vi "Begin.vi"(8 "error in":errorcluster) -> (0 "error out":errorcluster)   [LabVIEW 2015]
doc: "Called before other user functions, this VI is expected to open initial I/O refnums, load in file data, and do all program initialization. Notice that the <B>error out</B> terminal is simply used for data flow. Wiring it to other structures or subVIs ensures that this VI runs first."
uses:
  <vilib>/Rock Robotics/WPI/DriverStation/WPI_DriverStationRobotMode2.ctl
  <vilib>/Rock Robotics/WPI/Joystick/WPI_JoystickDeviceEnum.ctl
  <vilib>/Rock Robotics/SystemInterfaces/DIO/FPGA_DIOPWMChannel.ctl
  <vilib>/Rock Robotics/WPI/SafetyOutput/WPI_SafetyOutputConfigMenu.ctl
  <vilib>/Rock Robotics/WPI/Solenoid/WPI_SolenoidChannel.ctl
  <vilib>/Rock Robotics/SystemInterfaces/DIO/FPGA_DIOChannel.ctl
  <vilib>/Rock Robotics/WPI/Encoder/WPI_EncoderType.ctl
  <vilib>/Rock Robotics/SystemInterfaces/AI/FPGA_AIChannel.ctl
  <vilib>/Rock Robotics/SystemInterfaces/spilib/spi_bus.ctl
  Robot Global Data.vi
  <vilib>/Rock Robotics/WPI/Counter/WPI_CounterDigitalInputToDigitalSource.vi
  <vilib>/Rock Robotics/WPI/Solenoid/WPI_SolenoidOpenSingle.vi
  <vilib>/Rock Robotics/WPI/MotorControl/WPI_MotorControlOpen VictorSP.vi
  <vilib>/Rock Robotics/WPI/Utilities/WPI_GetSetVariantRefNum.vi
  navX Library v2/IO/Open/Z900_navX_Open_SPI.vi
  <vilib>/Rock Robotics/WPI/RobotDrive/WPI_RobotDriveOpen2MotorWithVictorSP.vi
  navX Library v2/navX Library v2.lvlib
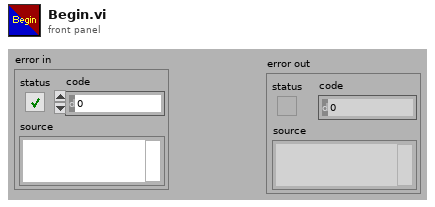
[diagram p1: front panel]
types:
  T1 = typedef "WPI_SolenoidChannel.ctl" = enum8{"Solenoid 0", "Solenoid 1", "Solenoid 2", "Solenoid 3", "Solenoid 4", "Solenoid 5", "Solenoid 6", "Solenoid 7", "Invalid"}
  T2 = typedef "FPGA_DIOPWMChannel.ctl" = enum8{"PWM 0", "PWM 1", "PWM 2", "PWM 3", "PWM 4", "PWM 5", "PWM 6", "PWM 7", "PWM 8", "PWM 9", "PWM MXP 0", "PWM MXP 1", "PWM MXP 2", "PWM MXP 3", "PWM MXP 4", "PWM MXP 5", "PWM MXP 6", "PWM MXP 7", "PWM MXP 8", "PWM MXP 9", "Invalid"}
  T3 = typedef "FPGA_DIOChannel.ctl" = enum8{"DIO 0", "DIO 1", "DIO 2", "DIO 3", "DIO 4", "DIO 5", "DIO 6", "DIO 7", "DIO 8", "DIO 9", "DIO MXP 0", "DIO MXP 1", "DIO MXP 2", "DIO MXP 3", "DIO MXP 4", "DIO MXP 5", "DIO MXP 6", "DIO MXP 7", "DIO MXP 8", "DIO MXP 9", "DIO MXP 10", "DIO MXP 11", "DIO MXP 12", "DIO MXP 13", "DIO MXP 14", "DIO MXP 15", "Invalid"}
  T4 = typedef "spi_bus.ctl" = enum16{"SPI On-Board, CS0", "SPI On-Board, CS1", "SPI On-Board, CS2", "SPI On-Board, CS3", "SPI MXP", "Invalid"}
  T5 = typedef "FPGA_AIChannel.ctl" = enum8{"AI 0", "AI 1", "AI 2", "AI 3", "AI MXP 0", "AI MXP 1", "AI MXP 2", "AI MXP 3", "Invalid"}
  T6 = typedef "WPI_JoystickDeviceEnum.ctl" = enum16{"USB 0", "USB 1", "USB 2", "USB 3", "USB 4", "USB 5"}
  T7 = typedef "WPI_EncoderType.ctl" = enum16{"1x", "2x", "4x"}
  T8 = typedef "WPI_SafetyOutputConfigMenu.ctl" = enum16{"Enable", "Disable"}
  T9 = typedef "WPI_DriverStationRobotMode2.ctl" = enum16{"Autonomous Disabled", "Autonomous Enabled", "Teleop Disabled", "Teleop Enabled", "Disconnected", "Finish", "Test Disabled", "Test Enabled", "Emergency Stopped"}
  T10 = typedef "WPI_MotorControlDeviceRef.ctl" = cluster{"DeviceStatus":errorcluster, "Type":T11, "PWM":cluster{"PWM Channel":T2, "DeadBand":T12}, "CAN":cluster{"Device Number":u8, "Control Mode":T13, "Semaphore":T14, "Max Vout":dbl, "TalonSRX Control Mode":T15}, "Invert":bool}
  T11 = typedef "WPI_MotorControlType.ctl" = enum16{"PWM", "CAN", "CANTalonSRX"}
  T12 = typedef "WPI_PWMDeadband.ctl" = cluster{"Name":string, "maxPositivePwm":i32, "minPositivePwm":i32, "centerPwm":i32, "maxNegativePwm":i32, "minNegativePwm":i32, "angularRange":u16}
  T13 = typedef "WPI_CANJaguar_ControlMode.ctl" = enum8{"Percent VBus", "Current", "Speed", "Position", "Voltage"}
  T14 = typedef "Semaphore RefNum" = refnum<k1>
  T15 = typedef "WPI_CANTalonSRX_APIControlMode.ctl" = enum8{"Percent VBus", "Speed", "Position", "Slave", "Unchanged / Invalid", "Voltage Compensation", "Current", "Motion Profile"}
  T16 = typedef "WPI_CompressorDevRef.ctl" = cluster{"DevStatus":errorcluster, "Pneumatics Control Module":u8}
  T17 = typedef "WPI_DigitalInputDevRef.ctl" = cluster{"DevStatus":errorcluster, "DIO Channel":T3}
  T18 = typedef "WPI_RobotDriveDevRef.ctl" = cluster{"DevStatus":errorcluster, "Motors[]":T10[], "Square Inputs":bool, "Max Output":dbl}
  T19 = typedef "WPI_JoystickDevRef.ctl" = cluster{"Device":T6}
  T20 = typedef "FPGA_CounterEncoderSourceConvertionLVSourceType.ctl" = cluster{"DevStatus":errorcluster, "AnalogTriggerMode?":bool, "DigitalMode":cluster{"DIO Channel":T21}, "AnalogTriggerMode":cluster{"AnalogTriggerIndex":T22, "OutputType":T23}}
  T21 = typedef "FPGA_DIODigitalSourceChannel.ctl" = enum8{"DIO 0", "DIO 1", "DIO 2", "DIO 3", "DIO 4", "DIO 5", "DIO 6", "DIO 7", "DIO 8", "DIO 9", "DIO MXP 0", "DIO MXP 1", "DIO MXP 2", "DIO MXP 3", "DIO MXP 4", "DIO MXP 5", "DIO MXP 6", "DIO MXP 7", "DIO MXP 8", "DIO MXP 9", "DIO MXP 10", "DIO MXP 11", "DIO MXP 12", "DIO MXP 13", "DIO MXP 14", "DIO MXP 15", "Disabled"}
  T22 = typedef "FPGA_AnalogTriggerIndex.ctl" = enum8{"Trig 0", "Trig 1", "Trig 2", "Trig 3", "Trig 4", "Trig 5", "Trig 6", "Trig 7", "Invalid"}
  T23 = typedef "FPGA_AnalogTriggerOutType.ctl" = enum16{"InWindow", "TriggerState", "Rising", "Falling"}
  T24 = typedef "navX Library v2.lvlib/Z900_navX_DeviceTypeDef.ctl" = cluster{"Interface":cluster{"Protocol":T25, "Update Rate (4Hz-60Hz)":u8, "navX Open TypeDef":variant}, "Notify Packet":refnum<notifier>, "Loop VI Refnum":refnum<vi>, "Ready to Close Occurrence Refnum":refnum<k4>}
  T25 = typedef "navX Library v2.lvlib/Z900_navX_ProtocolTypeDef.ctl" = enum16{"SERIAL", "I2C", "SPI"}
  T26 = typedef "WPI_AnalogChannelDevRef.ctl" = cluster{"DevStatus":errorcluster, "Analog Channel":T5}
  T27 = typedef "WPI_PotentiometerDevRef.ctl" = cluster{"DevStatus":errorcluster, "Analog Channel":T5, "Invert Output":bool}
  T28 = typedef "WPI_EncoderDevRef.ctl" = cluster{"DevStatus":errorcluster, "EncoderIndex":T29, "CounterIndex":T30, "DistancePerCount":dbl, "Decoding Type":T7}
  T29 = typedef "FPGA_EncoderIdx.ctl" = enum8{"Enc 0", "Enc 1", "Enc 2", "Enc 3", "Enc 4", "Enc 5", "Enc 6", "Enc 7", "Invalid"}
  T30 = typedef "FPGA_CounterCtrSystemIndex.ctl" = enum8{"Ctr 0", "Ctr 1", "Ctr 2", "Ctr 3", "Ctr 4", "Ctr 5", "Ctr 6", "Ctr 7", "Invalid"}
  T31 = typedef "WPI_SolenoidDevRef.ctl" = cluster{"DevStatus":errorcluster, "Pneumatics Control Module":u8, "Forward Solenoid Channel":T1, "Reverse Solenoid Channel":T1}
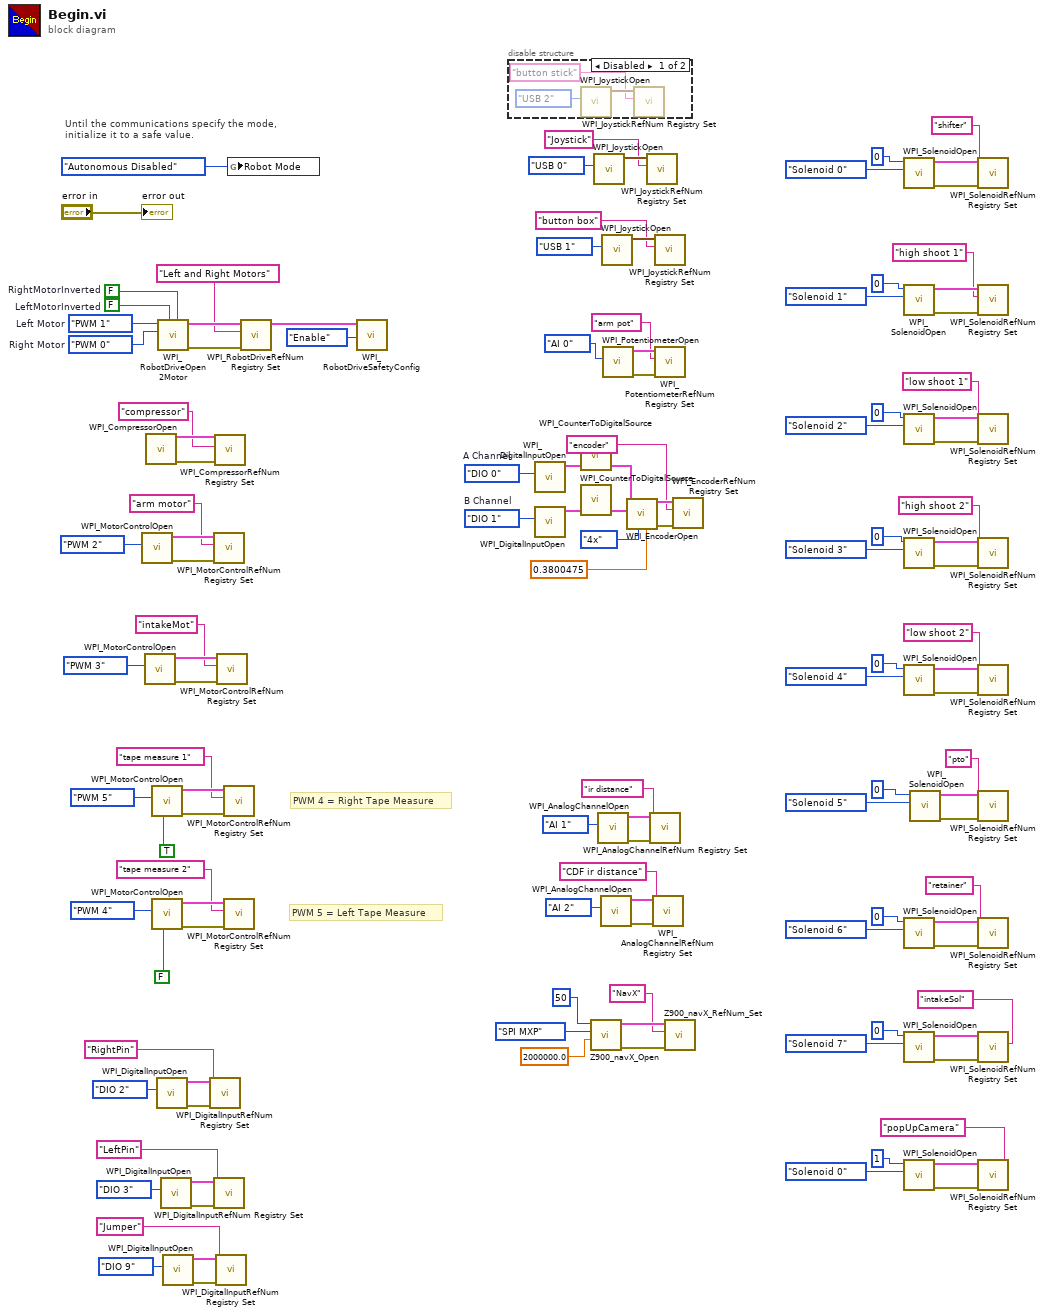
[diagram p0: block diagram]
diagram:
  w103 = FPGA_DIOChannel."DIO 1"  # B Channel
  w102 = FPGA_DIOChannel."DIO 0"  # A Channel
  w113 = FPGA_DIOPWMChannel."PWM 0"  # Right Motor
  w114 = FPGA_DIOPWMChannel."PWM 1"  # Left Motor
  w118 = FALSE  # LeftMotorInverted
  w119 = FALSE  # RightMotorInverted
  # "PWM 5 = Left Tape Measure"
  # "PWM 4 = Right Tape Measure"
  # "Until the communications specify the mode,\ninitialize it to a safe value."
  n1 = call-poly <vilib>:"WPI_MotorControlOpen.vi"("PWM Channel"=FPGA_DIOPWMChannel."PWM 2") -> ("error out"=w83:errorcluster, "MotorControlDeviceRef"=w82:T10)  [unwired: 9 in]
  n2 = call-poly <vilib>:"WPI_MotorControlOpen.vi"("PWM Channel"=FPGA_DIOPWMChannel."PWM 3") -> ("error out"=w59:errorcluster, "MotorControlDeviceRef"=w58:T10)  [unwired: 9 in]
  n3 = call <vilib>:"WPI_CompressorOpen.vi"() -> ("CompressorDevRef"=w105:T16, "error out"=w106:errorcluster)  [unwired: 14 in]
  n4 = call-poly <vilib>:"WPI_MotorControlOpen.vi"("Invert"=TRUE, "PWM Channel"=FPGA_DIOPWMChannel."PWM 5") -> ("error out"=w15:errorcluster, "MotorControlDeviceRef"=w14:T10)  [unwired: 8 in]
  n5 = call-poly <vilib>:"WPI_MotorControlOpen.vi"("Invert"=FALSE, "PWM Channel"=FPGA_DIOPWMChannel."PWM 4") -> ("error out"=w11:errorcluster, "MotorControlDeviceRef"=w10:T10)  [unwired: 8 in]
  n6 = call <vilib>:"WPI_DigitalInputOpen.vi"("DIO Channel"=FPGA_DIOChannel."DIO 2") -> ("error out"=w23:errorcluster, "DigitalInputDevRef"=w22:T17)  [unwired: 9 in]
  n7 = call-poly <vilib>:"WPI_RobotDriveOpen2Motor.vi"("Right Motor Inverted"=w119, "Left Motor Inverted"=w118, "Right Motor"=w113, "Left Motor"=w114) -> ("error out"=w115:errorcluster, "RobotDriveDevRef"=w117:T18)  [unwired: 1 in, 5 out]
  n8 = call <vilib>:"WPI_DigitalInputOpen.vi"("DIO Channel"=FPGA_DIOChannel."DIO 3") -> ("error out"=w19:errorcluster, "DigitalInputDevRef"=w18:T17)  [unwired: 9 in]
  n9 = call <vilib>:"WPI_DigitalInputOpen.vi"("DIO Channel"=FPGA_DIOChannel."DIO 9") -> ("error out"=w34:errorcluster, "DigitalInputDevRef"=w33:T17)  [unwired: 9 in]
  n10 = call <vilib>:"WPI_DigitalInputRefNum Registry Set.vi"("error in (no error)"=w23, "refnum name"="RightPin", "DigitalInputDevRef"=w22) -> ()  [unwired: 7 in, 2 out]
  n11 = call <vilib>:"WPI_MotorControlRefNum Registry Set.vi"("error in (no error)"=w83, "refnum name"="arm motor", "MotorControlDevRef"=w82) -> ()  [unwired: 7 in, 2 out]
  n12 = call <vilib>:"WPI_DigitalInputRefNum Registry Set.vi"("error in (no error)"=w19, "refnum name"="LeftPin", "DigitalInputDevRef"=w18) -> ()  [unwired: 7 in, 2 out]
  n13 = call <vilib>:"WPI_CompressorRefNum Registry Set.vi"("error in (no error)"=w106, "refnum name"="compressor", "CompressorDevRef"=w105) -> ()  [unwired: 7 in, 2 out]
  n14 = call <vilib>:"WPI_DigitalInputRefNum Registry Set.vi"("error in (no error)"=w34, "refnum name"="Jumper", "DigitalInputDevRef"=w33) -> ()  [unwired: 7 in, 2 out]
  n15 = call <vilib>:"WPI_MotorControlRefNum Registry Set.vi"("error in (no error)"=w59, "refnum name"="intakeMot", "MotorControlDevRef"=w58) -> ()  [unwired: 7 in, 2 out]
  n16 = call <vilib>:"WPI_MotorControlRefNum Registry Set.vi"("error in (no error)"=w15, "refnum name"="tape measure 1", "MotorControlDevRef"=w14) -> ()  [unwired: 7 in, 2 out]
  n17 = call <vilib>:"WPI_MotorControlRefNum Registry Set.vi"("error in (no error)"=w11, "refnum name"="tape measure 2", "MotorControlDevRef"=w10) -> ()  [unwired: 7 in, 2 out]
  n18 = global write "Robot Global Data.vi" "Robot Mode"(WPI_DriverStationRobotMode2."Autonomous Disabled" ("Robot Mode")) -> ()
  n19 = call <vilib>:"WPI_RobotDriveRefNum Registry Set.vi"("error in (no error)"=w115, "refnum name"="Left and Right Motors", "RobotDriveDevRef"=w117) -> ("RobotDriveDevRef"=w112:T18)  [unwired: 1 in, 7 out]
  n20 = call <vilib>:"WPI_RobotDriveSafetyConfig.vi"("mode"=WPI_SafetyOutputConfigMenu."Enable", "RobotDriveDevRef"=w112) -> ()  [unwired: 8 in, 2 out]
  n21 = disable-structure shown="Disabled" {
    frame Disabled {
      n22 = call <vilib>:"WPI_JoystickOpen.vi"("JoystickDevice"=WPI_JoystickDeviceEnum."USB 2") -> ("JoystickDevRef"=w127:T19)  [unwired: 10 in]
      n23 = call <vilib>:"WPI_JoystickRefNum Registry Set.vi"("refnum name"="button stick", "JoystickDevRef"=w127) -> ()  [unwired: 8 in, 2 out]
    }
    frame Enabled {
    }
  }
  n24 = call <vilib>:"WPI_DigitalInputOpen.vi"("DIO Channel"=w102) -> ("DigitalInputDevRef"=w99:T17)  [unwired: 1 in, 9 out]
  n25 = call <vilib>:"WPI_DigitalInputOpen.vi"("DIO Channel"=w103) -> ("DigitalInputDevRef"=w100:T17)  [unwired: 1 in, 9 out]
  n26 = call-poly <vilib>:"WPI_CounterToDigitalSource.vi"("DigitalInputDevRef"=w99) -> ("Digital Source"=w98:T20)  [unwired: 6 out]
  n27 = call-poly <vilib>:"WPI_CounterToDigitalSource.vi"("DigitalInputDevRef"=w100) -> ("Digital Source"=w101:T20)  [unwired: 6 out]
  n28 = call-poly "Z900_navX_Open.vi"("Clock Rate (Hz)"=2000000.0, "SPI Bus"=spi_bus."SPI MXP", "Update Rate (4Hz-60Hz)"=u8 50) -> ("error out"=w25:errorcluster, "navX Device"=w29:T24)  [unwired: 7 in]
  n29 = call <vilib>:"WPI_JoystickOpen.vi"("JoystickDevice"=WPI_JoystickDeviceEnum."USB 0") -> ("JoystickDevRef"=w122:T19)  [unwired: 10 in]
  n30 = call <vilib>:"WPI_AnalogChannelOpen.vi"("Analog Channel"=FPGA_AIChannel."AI 1") -> ("error out"=w50:errorcluster, "AIDeviceRef"=w49:T26)  [unwired: 9 in]
  n31 = call <vilib>:"WPI_AnalogChannelOpen.vi"("Analog Channel"=FPGA_AIChannel."AI 2") -> ("error out"=w38:errorcluster, "AIDeviceRef"=w37:T26)  [unwired: 9 in]
  n32 = call <vilib>:"WPI_JoystickOpen.vi"("JoystickDevice"=WPI_JoystickDeviceEnum."USB 1") -> ("JoystickDevRef"=w41:T19)  [unwired: 10 in]
  n33 = call <vilib>:"WPI_PotentiometerOpen.vi"("Analog Channel"=FPGA_AIChannel."AI 0") -> ("error out"=w87:errorcluster, "PotDevRef"=w86:T27)  [unwired: 9 in]
  n34 = call <vilib>:"WPI_EncoderOpen.vi"("DistancePerCount"=0.3800475, "Decoding Type"=WPI_EncoderType."4x", "BSource"=w101, "ASource"=w98) -> ("error out"=w96:errorcluster, "EncoderDevRef"=w97:T28)  [unwired: 4 in, 2 out]
  n35 = call <vilib>:"WPI_JoystickRefNum Registry Set.vi"("refnum name"="Joystick", "JoystickDevRef"=w122) -> ()  [unwired: 8 in, 2 out]
  n36 = call <vilib>:"WPI_AnalogChannelRefNum Registry Set.vi"("error in (no error)"=w50, "refnum name"="ir distance", "AIDeviceRef"=w49) -> ()  [unwired: 7 in, 2 out]
  n37 = call <vilib>:"WPI_AnalogChannelRefNum Registry Set.vi"("error in (no error)"=w38, "refnum name"="CDF ir distance", "AIDeviceRef"=w37) -> ()  [unwired: 7 in, 2 out]
  n38 = call <vilib>:"WPI_JoystickRefNum Registry Set.vi"("refnum name"="button box", "JoystickDevRef"=w41) -> ()  [unwired: 8 in, 2 out]
  n39 = call <vilib>:"WPI_PotentiometerRefNum Registry Set.vi"("error in (no error)"=w87, "refnum name"="arm pot", "PotDevRef"=w86) -> ()  [unwired: 7 in, 2 out]
  n40 = call "Z900_navX_RefNum_Set.vi"("error in (no error)"=w25, "refnum name"="NavX", "navX Device"=w29) -> ()  [unwired: 7 in, 2 out]
  n41 = call <vilib>:"WPI_EncoderRefNum Registry Set.vi"("error in (no error)"=w96, "refnum name"="encoder", "EncoderDevRef"=w97) -> ()  [unwired: 7 in, 2 out]
  n42 = call-poly <vilib>:"WPI_SolenoidOpen.vi"("Solenoid Channel"=WPI_SolenoidChannel."Solenoid 0", "Pneumatics Control Module (0)"=u8 0) -> ("error out"=w110:errorcluster, "SolenoidDevRef"=w109:T31)  [unwired: 8 in]
  n43 = call-poly <vilib>:"WPI_SolenoidOpen.vi"("Solenoid Channel"=WPI_SolenoidChannel."Solenoid 1", "Pneumatics Control Module (0)"=u8 0) -> ("error out"=w93:errorcluster, "SolenoidDevRef"=w92:T31)  [unwired: 8 in]
  n44 = call-poly <vilib>:"WPI_SolenoidOpen.vi"("Solenoid Channel"=WPI_SolenoidChannel."Solenoid 2", "Pneumatics Control Module (0)"=u8 0) -> ("error out"=w79:errorcluster, "SolenoidDevRef"=w78:T31)  [unwired: 8 in]
  n45 = call-poly <vilib>:"WPI_SolenoidOpen.vi"("Solenoid Channel"=WPI_SolenoidChannel."Solenoid 3", "Pneumatics Control Module (0)"=u8 0) -> ("error out"=w74:errorcluster, "SolenoidDevRef"=w73:T31)  [unwired: 8 in]
  n46 = call-poly <vilib>:"WPI_SolenoidOpen.vi"("Solenoid Channel"=WPI_SolenoidChannel."Solenoid 4", "Pneumatics Control Module (0)"=u8 0) -> ("error out"=w69:errorcluster, "SolenoidDevRef"=w68:T31)  [unwired: 8 in]
  n47 = call-poly <vilib>:"WPI_SolenoidOpen.vi"("Solenoid Channel"=WPI_SolenoidChannel."Solenoid 6", "Pneumatics Control Module (0)"=u8 0) -> ("error out"=w46:errorcluster, "SolenoidDevRef"=w45:T31)  [unwired: 8 in]
  n48 = call-poly <vilib>:"WPI_SolenoidOpen.vi"("Solenoid Channel"=WPI_SolenoidChannel."Solenoid 7", "Pneumatics Control Module (0)"=u8 0) -> ("error out"=w55:errorcluster, "SolenoidDevRef"=w54:T31)  [unwired: 8 in]
  n49 = call-poly <vilib>:"WPI_SolenoidOpen.vi"("Solenoid Channel"=WPI_SolenoidChannel."Solenoid 0", "Pneumatics Control Module (0)"=u8 1) -> ("error out"=w5:errorcluster, "SolenoidDevRef"=w4:T31)  [unwired: 8 in]
  n50 = call-poly <vilib>:"WPI_SolenoidOpen.vi"("Solenoid Channel"=WPI_SolenoidChannel."Solenoid 5", "Pneumatics Control Module (0)"=u8 0) -> ("error out"=w64:errorcluster, "SolenoidDevRef"=w63:T31)  [unwired: 8 in]
  n51 = call <vilib>:"WPI_SolenoidRefNum Registry Set.vi"("error in (no error)"=w110, "refnum name"="shifter", "SolenoidDevRef"=w109) -> ()  [unwired: 7 in, 2 out]
  n52 = call <vilib>:"WPI_SolenoidRefNum Registry Set.vi"("error in (no error)"=w93, "refnum name"="high shoot 1", "SolenoidDevRef"=w92) -> ()  [unwired: 7 in, 2 out]
  n53 = call <vilib>:"WPI_SolenoidRefNum Registry Set.vi"("error in (no error)"=w79, "refnum name"="low shoot 1", "SolenoidDevRef"=w78) -> ()  [unwired: 7 in, 2 out]
  n54 = call <vilib>:"WPI_SolenoidRefNum Registry Set.vi"("error in (no error)"=w74, "refnum name"="high shoot 2", "SolenoidDevRef"=w73) -> ()  [unwired: 7 in, 2 out]
  n55 = call <vilib>:"WPI_SolenoidRefNum Registry Set.vi"("error in (no error)"=w69, "refnum name"="low shoot 2", "SolenoidDevRef"=w68) -> ()  [unwired: 7 in, 2 out]
  n56 = call <vilib>:"WPI_SolenoidRefNum Registry Set.vi"("error in (no error)"=w64, "refnum name"="pto", "SolenoidDevRef"=w63) -> ()  [unwired: 7 in, 2 out]
  n57 = call <vilib>:"WPI_SolenoidRefNum Registry Set.vi"("error in (no error)"=w46, "refnum name"="retainer", "SolenoidDevRef"=w45) -> ()  [unwired: 7 in, 2 out]
  n58 = call <vilib>:"WPI_SolenoidRefNum Registry Set.vi"("error in (no error)"=w55, "refnum name"="intakeSol", "SolenoidDevRef"=w54) -> ()  [unwired: 7 in, 2 out]
  n59 = call <vilib>:"WPI_SolenoidRefNum Registry Set.vi"("error in (no error)"=w5, "refnum name"="popUpCamera", "SolenoidDevRef"=w4) -> ()  [unwired: 7 in, 2 out]
  "error out" <- "error in"
